vi "Wait for hexapod system axes to stop.vi"(0 "System no.":i32=1, 2 "Axes to wait for":string[](array[string]), 3 "All axes?":bool=TRUE, 5 "error in":errorcluster, 12 "Stop refnum":refnum<vi>) -> (14 "Stopped":bool, 19 "error out":errorcluster)   [LabVIEW 2026]
doc: "This VI waits for the specified axes of a PI hexapod system (hexapod axes X, Y, Z, U, V, W and separate axes A, B) to stop using #5 polling. If a NanoCube axis (K, L or M) is commanded, the VI will return immediately. If one of the hexapod axes (X, Y, Z, U, V or W) is commanded, it will wait for all six hexapod axes to stop. It returns immediately if a communications error occured, or if Stop refnum or Local stop is TRUE. When using as a sub-VI, use Stop refnum to stop VI from caller. Required by General wait for movement to stop.vi.\n\nTo wait for the hexapod to stop, only one hexapod axis (X, Y, Z, U, V or W) needs to be commanded, because the VI cannot distinguish between the different hexapod axes. \n\nC-887, F-206: Axes to wait for can be any of X, Y, Z, U, V, W, A, B, K, L, M\nM-8X0: Axes to wait for can be any of X, Y, Z, U, V, W, A, B"
panel:
  in  "Local stop":bool
  # "This vi waits for the specified axes of a PI hexapod system\n(F-206, M-840, M-850) to stop using #5 polling. It returns\nimmediately if a communications error occured, or if Stop \nrefnum or Local stop is TRUE. See manual for further explanation."
  # "Wait for"
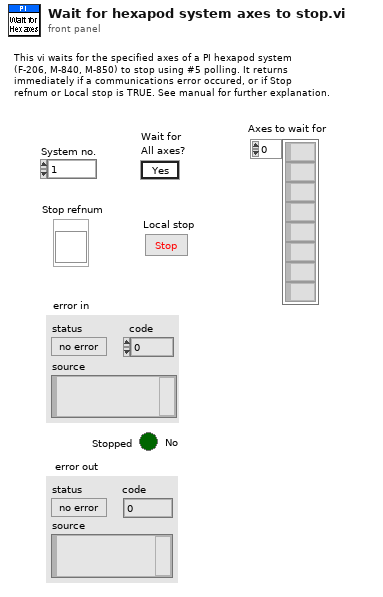
[diagram p1: front panel]
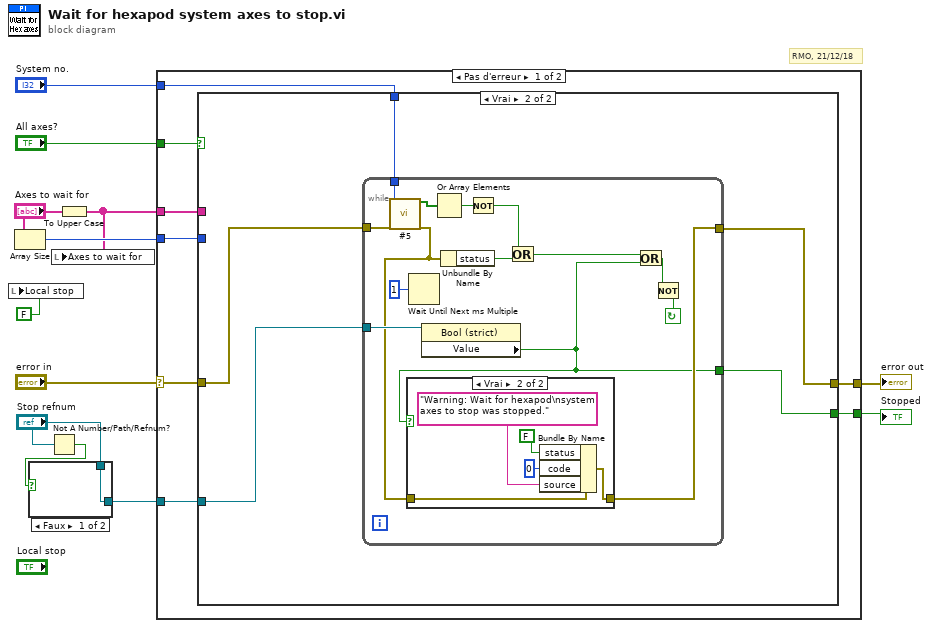
[diagram p0: block diagram]
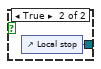
[diagram p2: hidden frame]
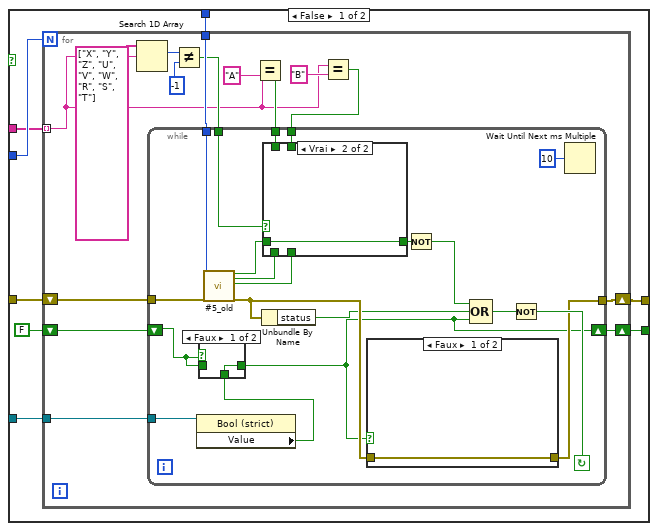
[diagram p3: hidden frame]
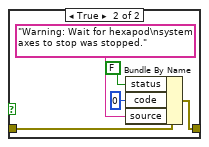
[diagram p5: hidden frame]
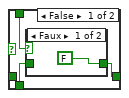
[diagram p7: hidden frame]
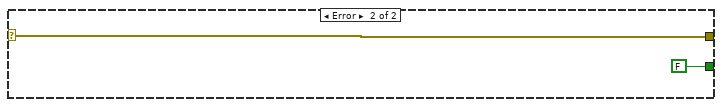
[diagram p10: hidden frame]
diagram:
  # "RMO, 21/12/18"
  n1 = local write "Local stop"(FALSE ("Local stop")) -> ()
  n2 = Array Size(array="Axes to wait for") -> (size(s)=w10:i32)
  n3 = Not A Number/Path/Refnum?(number/path/refnum="Stop refnum") -> (NaN/Path/Refnum?=w5:bool)
  n4 = case shown="Faux" w5 {
    tunnel: [w13 w14] -> w3
    tunnel: "Stop refnum" -> [w13 _]
    frame False {
    }
    frame True {
      n5 = control-ref of="Local stop"() -> (w14:refnum<vi>)
    }
  }
  n6 = To Upper Case(1:"Axes to wait for") -> (0:w8:string[])
  n7 = local write "Axes to wait for"(w8) -> ()
  n8 = case shown="Pas d'erreur" "error in" {
    selector: "error in" -> [w15 w111]
    tunnel: "System no." -> [w22 _]
    tunnel: w8 -> [w18 _]
    tunnel: w10 -> [w19 _]
    tunnel: [w21 w111] -> w9
    tunnel: "All axes?" -> [w20 _]
    tunnel: w3 -> [w17 _]
    tunnel: [w16 FALSE ("Value")] -> w2
    frame No Error {
      n9 = case shown="Vrai" w20 {
        tunnel: w22 -> [w28 w88]
        tunnel: [w26 w90] -> w21
        tunnel: w15 -> [w27 w89]
        tunnel: w19 -> [w30 _]
        tunnel: w18 -> [w29 _]
        tunnel: w17 -> [w25 w87]
        tunnel: [w24 w86] -> w16
        frame False {
          n10 = for {
            N: w30 -> [_]
            tunnel: w29 -> [w37] mode=indexing
            tunnel: w28 -> [w42]
            shift-right: [w34] -> w26
            shift-left: w27 -> [w35]
            tunnel: w25 -> [w33]
            shift-right: [w31] -> w24
            shift-left: FALSE ("Value") -> [w32]
            n11 = Search 1D Array(1D array=string[] ["X", "Y", "Z", "U", "V", "W", "R", "S", "T"] ("Conn. axes"), element=w37) -> (index of element=w44:i32)  [unwired: 1 out]
            n12 = Not Equal?(x=w44, y=-1) -> (x != y?=w39:bool)
            n13 = Equal?(x=w37, y="A") -> (x = y?=w38:bool)
            n14 = Equal?(x=w37, y="B") -> (x = y?=w36:bool)
            n15 = while {
              shift-left: w32 -> [w47]
              shift-right: [w46] -> w31
              tunnel: w33 -> [w52]
              tunnel: w36 -> [w58]
              tunnel: w38 -> [w60]
              tunnel: w39 -> [w61]
              tunnel: [w54] -> w34
              tunnel: w35 -> [w64]
              tunnel: w42 -> [w63]
              stop <- w55 continue-if-true
              n16 = property class="Bool (strict)"(reference=w52) -> ("Value"=w48:bool)  [unwired: 1 in, 2 out]
              n17 = case shown="Faux" w47 {
                tunnel: [w66 w67] -> w46
                tunnel: w47 -> [_ w67]
                tunnel: w48 -> [w66 _]
                frame False {
                }
                frame True {
                }
              }
              n18 = call "#5_old.vi"("System no."=w63, "error in"=w64) -> ("Overall system\nmoving?"=w62:bool, "Sep. Axis 1\nmoving?"=w59:bool, "Sep. Axis 2\nmoving?"=w57:bool, "error out"=w53:errorcluster)  [unwired: 14 out]
              n19 = Unbundle By Name(w53) -> ("status"=w51:bool)
              n20 = case shown="Vrai" w61 {
                tunnel: [w76 w85] -> w50
                tunnel: w62 -> [_ w85]
                tunnel: w60 -> [w78 _]
                tunnel: w59 -> [w77 _]
                tunnel: w58 -> [w75 _]
                tunnel: w57 -> [w74 _]
                frame False {
                  n21 = case shown="Vrai" w78 {
                    tunnel: w77 -> [_ w84]
                    tunnel: [w79 w84] -> w76
                    tunnel: w75 -> [w81 _]
                    tunnel: w74 -> [w80 _]
                    frame False {
                      n22 = case shown="Faux" w81 {
                        tunnel: w80 -> [_ w83]
                        tunnel: [FALSE ("Sep. Axis 2\nmoving?") w83] -> w79
                        frame False {
                        }
                        frame True {
                        }
                      }
                    }
                    frame True {
                    }
                  }
                }
                frame True {
                }
              }
              n23 = case shown="Faux" w46 {
                tunnel: w53 -> [w68 w69]
                tunnel: [w68 w70] -> w54
                frame False {
                }
                frame True {
                  n24 = Bundle By Name(cluster=w69, "status"=FALSE, "code"=0, "source"="Warning: Wait for hexapod\nsystem axes to stop was stopped.") -> (w70:errorcluster)
                }
              }
              n25 = Not(x=w50) -> (.not. x?=w49:bool)
              n26 = Compound Arithmetic op=OR(w49, w51, w46) -> (w56:bool)
              n27 = Not(x=w56) -> (.not. x?=w55:bool)
              n28 = Wait Until Next ms Multiple(millisecond multiple=u32 10) -> ()  [unwired: 1 out]
            }
          }
        }
        frame True {
          n29 = while {
            tunnel: [w91] -> w86
            tunnel: w87 -> [w96]
            tunnel: [w92] -> w90
            tunnel: w89 -> [w103]
            tunnel: w88 -> [w102]
            stop <- w94 continue-if-true
            n30 = call "#5.vi"("System no."=w102, "error in"=w103) -> ("Axis moving?"=w101:bool[], "error out"=w93:errorcluster)  [unwired: 16 out]
            n31 = Wait Until Next ms Multiple(millisecond multiple=u32 1) -> ()  [unwired: 1 out]
            n32 = property class="Bool (strict)"(reference=w96) -> ("Value"=w91:bool)  [unwired: 1 in, 2 out]
            n33 = case shown="Vrai" w91 {
              tunnel: w93 -> [w105 w106]
              tunnel: [w105 w107] -> w92
              frame False {
              }
              frame True {
                n34 = Bundle By Name(cluster=w106, "status"=FALSE, "code"=0, "source"="Warning: Wait for hexapod\nsystem axes to stop was stopped.") -> (w107:errorcluster)
              }
            }
            n35 = Or Array Elements(Boolean array=w101) -> (logical OR=w100:bool)
            n36 = Unbundle By Name(w93) -> ("status"=w99:bool)
            n37 = Not(x=w100) -> (.not. x?=w98:bool)
            n38 = Or(x=w98, y=w99) -> (x .or. y?=w97:bool)
            n39 = Or(x=w97, y=w91) -> (x .or. y?=w95:bool)
            n40 = Not(x=w95) -> (.not. x?=w94:bool)
          }
        }
      }
    }
    frame Error {
    }
  }
  "error out" <- w9
  "Stopped" <- w2
